vi "Set T-time.vi"(6 "errorIN":errorcluster caption="Error In", 8 "Count Time Set":dbl[unit], 9 "VISA resource name":refnum<visa-resource-name>) -> (0 "errorOUT":errorcluster caption="Error Out", 2 "ttimeOUT":dbl[unit]=1.0 caption="Count Time Current" min=0.0 max=10000.0 step=1.0 format="%#_7g", 3 "VISA resource name out":refnum<visa-resource-name>)   [LabVIEW 2015, in "SR400.lvlib"]
uses:
  SR400.lvlib
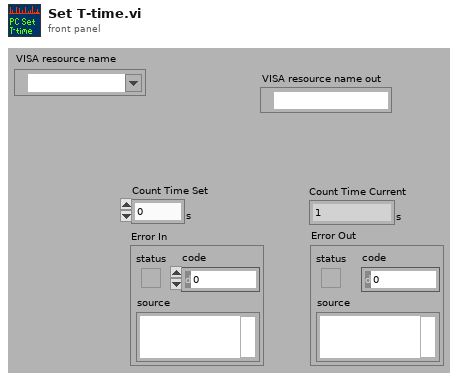
[diagram p1: front panel]
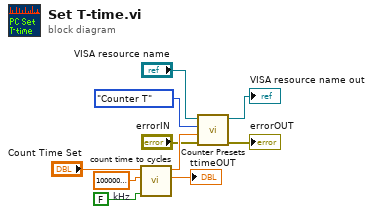
[diagram p0: block diagram]
diagram:
  w9 = dbl[unit] 10000000.0  # kHz
  n1 = call "count time to cycles.vi"("dispmsg?"=FALSE, "Trigger Freq"=w9, "Count Time Set"="Count Time Set") -> ("Count Time Current"=→"ttimeOUT":dbl[unit], "Number of triggers"=w5:dbl)  [unwired: 3 out]
  n2 = call "Counter Presets.vi"("error in (no error)"="errorIN", "Number of triggers"=w5, "Counter (Def: T)"=enum16{"Invalid", "Counter B", "Counter T"}."Counter T" ("i (0) 2"), "VISA resource name"="VISA resource name") -> ("error out"=→"errorOUT":errorcluster, "VISA resource name out"=→"VISA resource name out":refnum<visa-resource-name>)  [unwired: 6 out]
